vi "读取-剂量率.vi"(8 "error in (no error)":errorcluster caption="错误输入（无错误）", 11 "设备终端输入":refnum<class "设备终端.lvclass">) -> (0 "error out":errorcluster caption="错误输出", 2 "剂量率":cluster{"剂量率":dbl, "时间":timestamp}, 3 "设备终端输出":refnum<class "设备终端.lvclass">)   [LabVIEW 2013, in "设备终端.lvclass"]
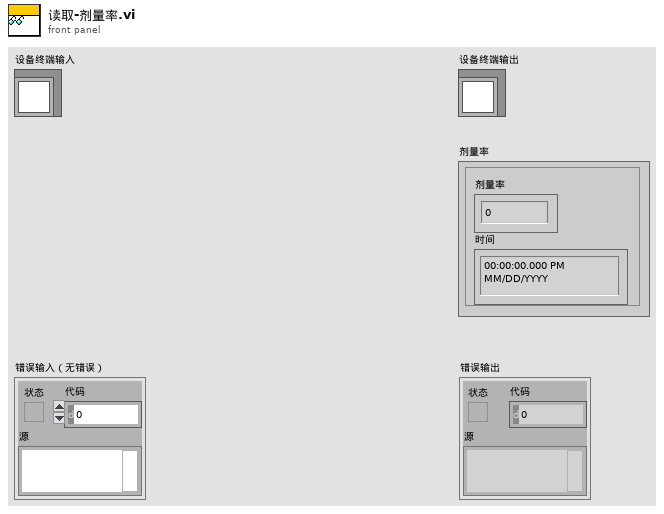
[diagram p1: front panel]
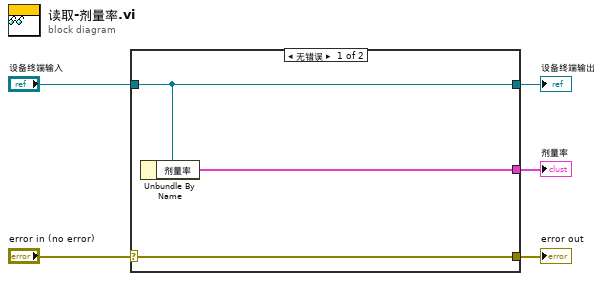
[diagram p0: block diagram]
diagram:
  n1 = case shown="无错误" "error in (no error)" {
    selector: "error in (no error)" -> [w8 w9]
    tunnel: [w8 w9] -> w4
    tunnel: [w7 w10] -> w2
    tunnel: "设备终端输入" -> [w7 w10]
    tunnel: [w6 _] -> w1
    frame No Error {
      n2 = Unbundle By Name(w7) -> ("剂量率"=w6:cluster{"剂量率":dbl, "时间":timestamp})
    }
    frame Error {
    }
  }
  "error out" <- w4
  "设备终端输出" <- w2
  "剂量率" <- w1
